vi "MatrixToString.vi"(10 "Header (default: no header)":string, 11 "Matrix in":T1) -> (3 "String out":string)   [LabVIEW 2014, in "Supervisor.lvclass"]
uses:
  Supervisor/Supervisor.lvclass
  <vilib>/Analysis/Matrix/Datatypes/RealMatrix.ctl
  <vilib>/Analysis/Matrix/NI_Matrix.lvlib
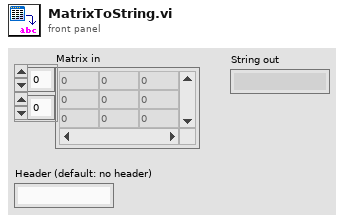
[diagram p1: front panel]
types:
  T1 = typedef "NI_Matrix.lvlib/RealMatrix.ctl" = dbl[][]
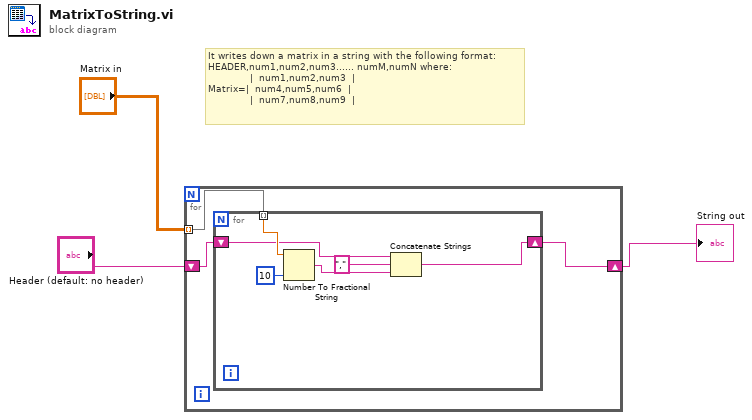
[diagram p0: block diagram]
diagram:
  # "It writes down a matrix in a string with the following format:\nHEADER,num1,num2,num3...... numM,numN where:\n              |  num1,num2,num3  |\nMatrix=|  num4,num5,num6  |\n              |  num7,num8,num9  |"
  n1 = for {
    shift-right: [w6] -> w1
    shift-left: "Header (default: no header)" -> [w5]
    tunnel: "Matrix in" -> [w4] mode=indexing
    n2 = for {
      shift-right: [w10] -> w6
      shift-left: w5 -> [w11]
      tunnel: w4 -> [w12] mode=indexing
      n3 = Number To Fractional String(number=w12, precision (6)=i16 10) -> (F-format string=w9:string)  [unwired: 2 in]
      n4 = Concatenate Strings(w11, "," ("String"), w9) -> (w10:string)
    }
  }
  "String out" <- w1
